vi "Lift Cases.vi"() -> ()   [LabVIEW 2014]
uses:
  Begin/Global Variables.vi
panel:
  in  "Lift Speed":dbl=1.0 format="%#_13g"
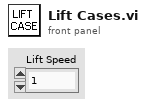
[diagram p1: front panel]
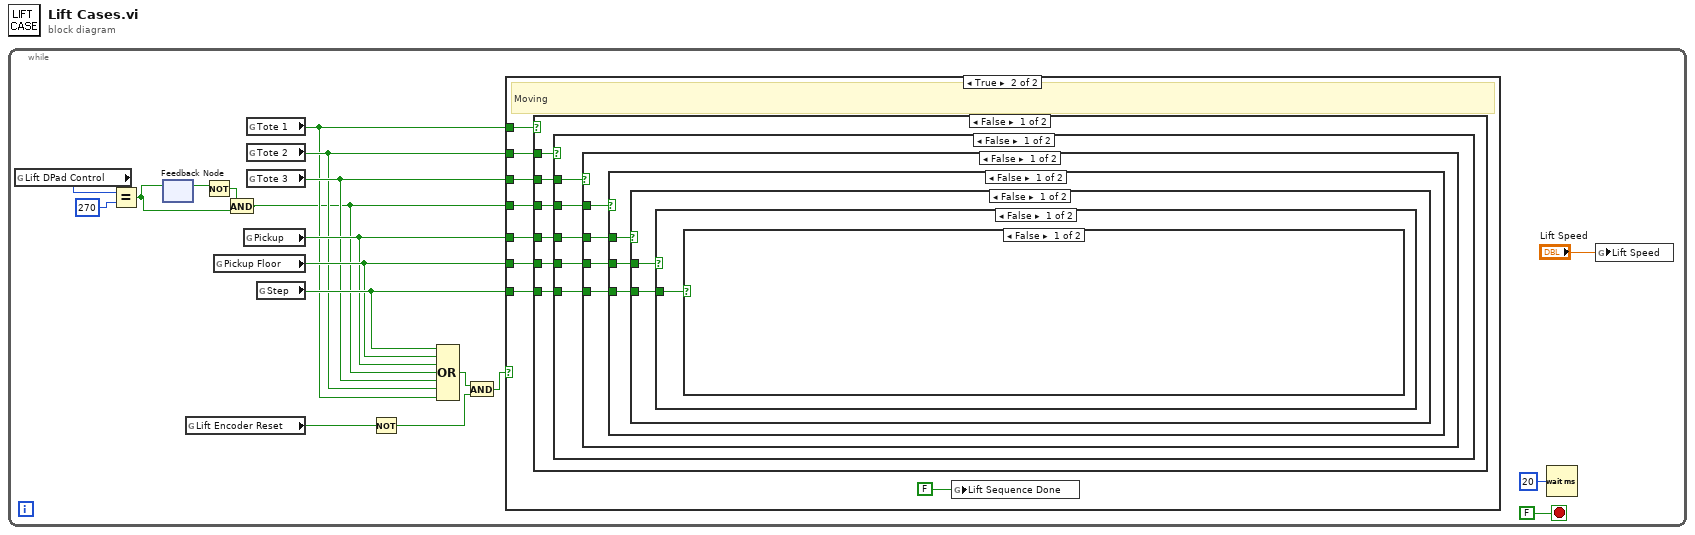
[diagram p0: block diagram]
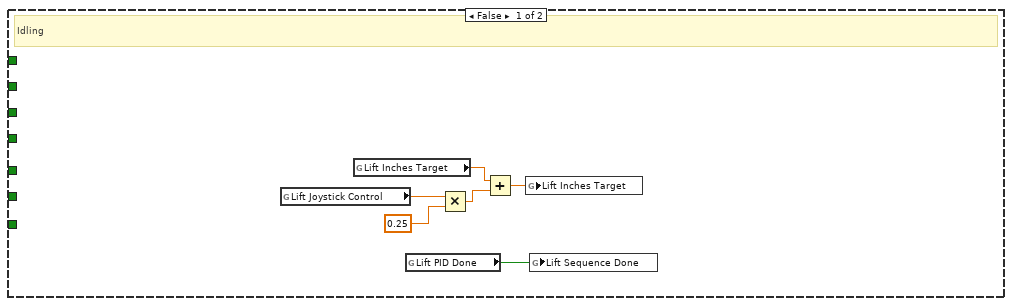
[diagram p2: hidden frame]
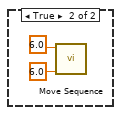
[diagram p3: hidden frame]
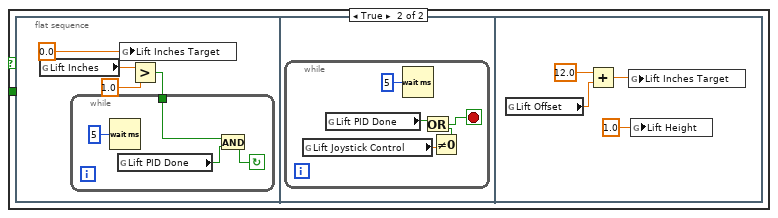
[diagram p4: hidden frame]
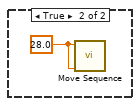
[diagram p5: hidden frame]
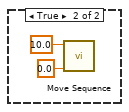
[diagram p6: hidden frame]
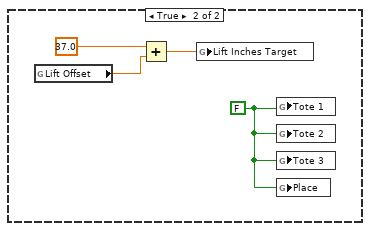
[diagram p7: hidden frame]
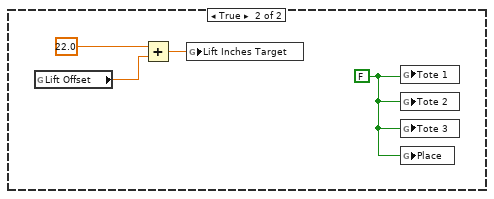
[diagram p8: hidden frame]
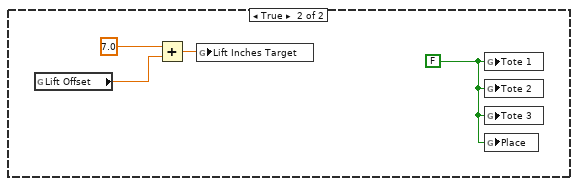
[diagram p9: hidden frame]
diagram:
  n1 = while {
    stop <- FALSE stop-if-true
    n2 = global read "Global Variables.vi" "Lift DPad Control"() -> (w1:i16)
    n3 = Equal?(x=w1, y=i16 270) -> (x = y?=w6:bool)
    n4 = feedback #1() -> (w5:bool)  [unwired: 1 in]
    n5 = feedback-in #1(w6) -> ()
    n6 = global read "Global Variables.vi" "Lift Encoder Reset"() -> (w9:bool)
    n7 = Not(x=w5) -> (.not. x?=w4:bool)
    n8 = global read "Global Variables.vi" "Pickup Floor"() -> (w16:bool)
    n9 = And(x=w4, y=w6) -> (x .and. y?=w2:bool)
    n10 = global read "Global Variables.vi" "Pickup"() -> (w15:bool)
    n11 = global read "Global Variables.vi" "Tote 1"() -> (w12:bool)
    n12 = global read "Global Variables.vi" "Tote 2"() -> (w13:bool)
    n13 = global read "Global Variables.vi" "Tote 3"() -> (w14:bool)
    n14 = global read "Global Variables.vi" "Step"() -> (w17:bool)
    n15 = Not(x=w9) -> (.not. x?=w8:bool)
    n16 = Compound Arithmetic op=OR(w17, w16, w15, w2, w14, w13, w12) -> (w10:bool)
    n17 = And(x=w10, y=w8) -> (x .and. y?=w7:bool)
    n18 = case shown="True" w7 {
      tunnel: w12 -> [_ w33]
      tunnel: w13 -> [_ w32]
      tunnel: w14 -> [_ w31]
      tunnel: w2 -> [_ w30]
      tunnel: w15 -> [_ w29]
      tunnel: w16 -> [_ w28]
      tunnel: w17 -> [_ w27]
      frame False {
        # "Idling"
        n19 = global read "Global Variables.vi" "Lift Joystick Control"() -> (w21:dbl)
        n20 = global read "Global Variables.vi" "Lift Inches Target"() -> (w23:dbl)
        n21 = global read "Global Variables.vi" "Lift PID Done"() -> (w25:bool)
        n22 = Multiply(x=w21, y=0.25) -> (x*y=w22:dbl)
        n23 = Add(x=w23, y=w22) -> (x+y=w24:dbl)
        n24 = global write "Global Variables.vi" "Lift Inches Target"(w24) -> ()
        n25 = global write "Global Variables.vi" "Lift Sequence Done"(w25) -> ()
      }
      frame True {
        # "Moving"
        n26 = case shown="False" w33 {
          tunnel: w32 -> [w39 _]
          tunnel: w31 -> [w38 _]
          tunnel: w30 -> [w37 _]
          tunnel: w29 -> [w36 _]
          tunnel: w28 -> [w35 _]
          tunnel: w27 -> [w34 _]
          frame False {
            n27 = case shown="False" w39 {
              tunnel: w38 -> [w44 _]
              tunnel: w37 -> [w43 _]
              tunnel: w36 -> [w42 _]
              tunnel: w35 -> [w41 _]
              tunnel: w34 -> [w40 _]
              frame False {
                n28 = case shown="False" w44 {
                  tunnel: w43 -> [w48 _]
                  tunnel: w42 -> [w47 _]
                  tunnel: w41 -> [w46 _]
                  tunnel: w40 -> [w45 _]
                  frame False {
                    n29 = case shown="False" w48 {
                      tunnel: w47 -> [w51 _]
                      tunnel: w46 -> [w50 _]
                      tunnel: w45 -> [w49 _]
                      frame False {
                        n30 = case shown="False" w51 {
                          tunnel: w50 -> [w53 _]
                          tunnel: w49 -> [w52 _]
                          frame False {
                            n31 = case shown="False" w53 {
                              tunnel: w52 -> [w54 _]
                              frame False {
                                n32 = case shown="False" w54 {
                                frame False {
                                }
                                frame True {
                                n33 = call "Move Sequence.vi"("Distance Up"=6.0, "Distance Down"=6.0) -> ()  [unwired: 10 in]
                                }
                                }
                              }
                              frame True {
                                n34 = flat-sequence {
                                frame #0 {
                                n35 = global read "Global Variables.vi" "Lift Inches"() -> (w58:dbl)
                                n36 = global write "Global Variables.vi" "Lift Inches Target"(0.0 ("x")) -> ()
                                n37 = Greater?(x=w58, y=1.0) -> (0:w57:bool)
                                n38 = while {
                                tunnel: w57 -> [w61]
                                stop <- w62 continue-if-true
                                n39 = Wait (ms)(milliseconds to wait=u32 5) -> ()  [unwired: 1 out]
                                n40 = global read "Global Variables.vi" "Lift PID Done"() -> (w63:bool)
                                n41 = And(x=w61, y=w63) -> (x .and. y?=w62:bool)
                                }
                                }
                                frame #1 {
                                n42 = while {
                                stop <- w65 stop-if-true
                                n43 = global read "Global Variables.vi" "Lift Joystick Control"() -> (w68:dbl)
                                n44 = global read "Global Variables.vi" "Lift PID Done"() -> (w66:bool)
                                n45 = Wait (ms)(milliseconds to wait=u32 5) -> ()  [unwired: 1 out]
                                n46 = Not Equal To 0?(x=w68) -> (x != 0?=w67:bool)
                                n47 = Or(x=w66, y=w67) -> (x .or. y?=w65:bool)
                                }
                                }
                                frame #2 {
                                n48 = global read "Global Variables.vi" "Lift Offset"() -> (w70:dbl)
                                n49 = Add(x=12.0, y=w70) -> (x+y=w72:dbl)
                                n50 = global write "Global Variables.vi" "Lift Inches Target"(w72) -> ()
                                n51 = global write "Global Variables.vi" "Lift Height"(1.0 ("Lift Height")) -> ()
                                }
                                }
                              }
                            }
                          }
                          frame True {
                            w74 = 28.0 ("Distance Down")
                            n52 = call "Move Sequence.vi"("Distance Up"=w74, "Distance Down"=w74) -> ()  [unwired: 10 in]
                          }
                        }
                      }
                      frame True {
                        n53 = call "Move Sequence.vi"("Distance Up"=0.0, "Distance Down"=10.0 ("Distance Down 2")) -> ()  [unwired: 10 in]
                      }
                    }
                  }
                  frame True {
                    w77 = FALSE ("Tote 0")
                    n54 = global read "Global Variables.vi" "Lift Offset"() -> (w78:dbl)
                    n55 = Add(x=37.0 ("x 3"), y=w78) -> (x+y=w79:dbl)
                    n56 = global write "Global Variables.vi" "Lift Inches Target"(w79) -> ()
                    n57 = global write "Global Variables.vi" "Tote 1"(w77) -> ()
                    n58 = global write "Global Variables.vi" "Tote 2"(w77) -> ()
                    n59 = global write "Global Variables.vi" "Tote 3"(w77) -> ()
                    n60 = global write "Global Variables.vi" "Place"(w77) -> ()
                  }
                }
              }
              frame True {
                w81 = FALSE ("Tote 0")
                n61 = global read "Global Variables.vi" "Lift Offset"() -> (w82:dbl)
                n62 = Add(x=22.0 ("x 2"), y=w82) -> (x+y=w83:dbl)
                n63 = global write "Global Variables.vi" "Lift Inches Target"(w83) -> ()
                n64 = global write "Global Variables.vi" "Tote 1"(w81) -> ()
                n65 = global write "Global Variables.vi" "Tote 2"(w81) -> ()
                n66 = global write "Global Variables.vi" "Tote 3"(w81) -> ()
                n67 = global write "Global Variables.vi" "Place"(w81) -> ()
              }
            }
          }
          frame True {
            w85 = FALSE ("Tote 0")
            n68 = global read "Global Variables.vi" "Lift Offset"() -> (w86:dbl)
            n69 = Add(x=7.0, y=w86) -> (x+y=w87:dbl)
            n70 = global write "Global Variables.vi" "Lift Inches Target"(w87) -> ()
            n71 = global write "Global Variables.vi" "Tote 1"(w85) -> ()
            n72 = global write "Global Variables.vi" "Tote 2"(w85) -> ()
            n73 = global write "Global Variables.vi" "Tote 3"(w85) -> ()
            n74 = global write "Global Variables.vi" "Place"(w85) -> ()
          }
        }
        n75 = global write "Global Variables.vi" "Lift Sequence Done"(FALSE ("Lift Sequence Done")) -> ()
      }
    }
    n76 = Wait (ms)(milliseconds to wait=u32 20) -> ()  [unwired: 1 out]
    n77 = global write "Global Variables.vi" "Lift Speed"("Lift Speed") -> ()
  }
